vi "Read Stored State DVR.vi"(8 "error in (no error)":errorcluster, 11 "Collect Data in":refnum<class "Collect Data.lvclass">) -> (0 "error out":errorcluster, 2 "Stored State DVR":refnum<data-value>, 3 "Collect Data out":refnum<class "Collect Data.lvclass">)   [LabVIEW 2015, in "Collect Data.lvclass"]
uses:
  Collect Data.lvclass
  State data/State Data.lvclass
  Collect Data.lvclass/Collect Data.ctl
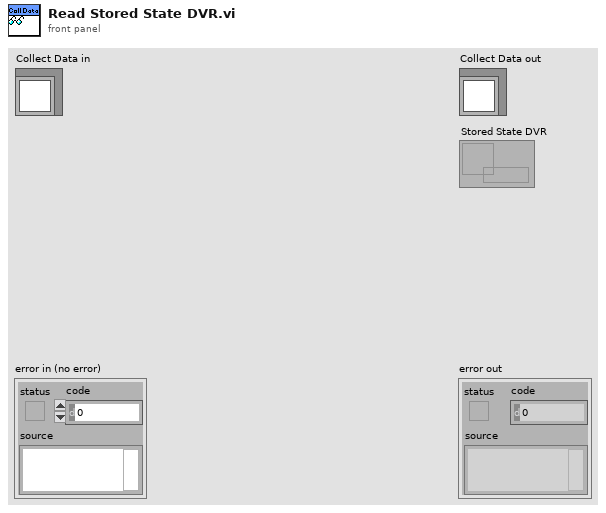
[diagram p1: front panel]
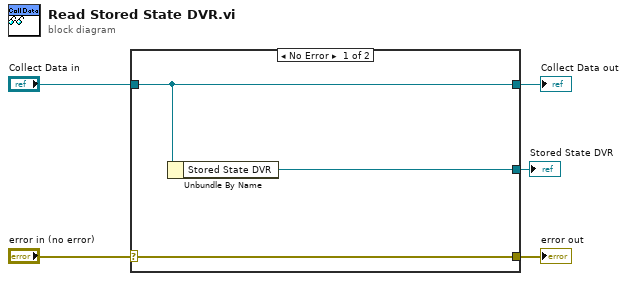
[diagram p0: block diagram]
diagram:
  n1 = case shown="No Error" "error in (no error)" {
    selector: "error in (no error)" -> [w8 w9]
    tunnel: [w8 w9] -> w4
    tunnel: [w7 w10] -> w2
    tunnel: "Collect Data in" -> [w7 w10]
    tunnel: [w6 _] -> w1
    frame No Error {
      n2 = Unbundle By Name(w7) -> ("Stored State DVR"=w6:refnum<data-value>)
    }
    frame Error {
    }
  }
  "error out" <- w4
  "Collect Data out" <- w2
  "Stored State DVR" <- w1
